vi "Set Component Licenses.vi"(8 "error in (no error)":errorcluster, 10 "License(s)":refnum<class "CycloneDX License.lvclass">[](array[class]), 11 "CycloneDX Component in":refnum<class "CycloneDX Component.lvclass">) -> (0 "error out":errorcluster, 3 "CycloneDX Component out":refnum<class "CycloneDX Component.lvclass">)   [LabVIEW 2017, in "LabVIEW CycloneDX SBOM.lvlib" / "CycloneDX Component.lvclass"]
uses:
  CycloneDX Component.lvclass
  C:/LabVIEW Working Directory/labview-cyclonedx-sbom/Source/CycloneDX/CycloneDX JSON/CycloneDX JSON.lvclass
  CycloneDX License/CycloneDX License.lvclass
  CycloneDX JSON/CycloneDX JSON.lvclass/CycloneDX JSON.ctl
  CycloneDX JSON/Read JSON.vi
  <vilib>/JDP Science/JSONtext/support/Format JSON Array Text.vi
  CycloneDX JSON/CycloneDX JSON.lvclass
  <vilib>/JDP Science/JSONtext/JSONtext.lvlib
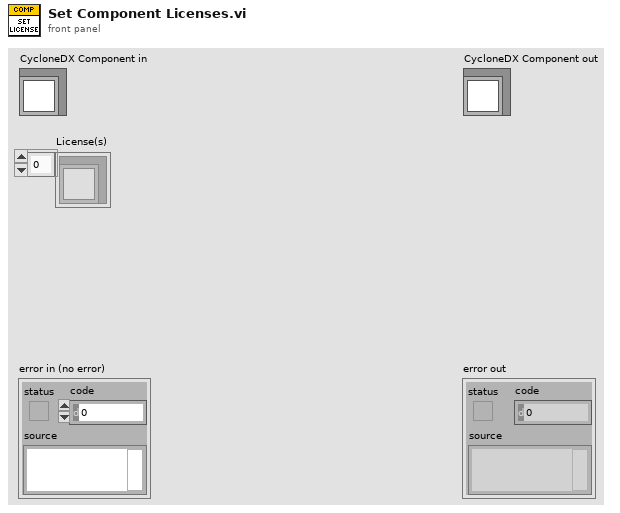
[diagram p1: front panel]
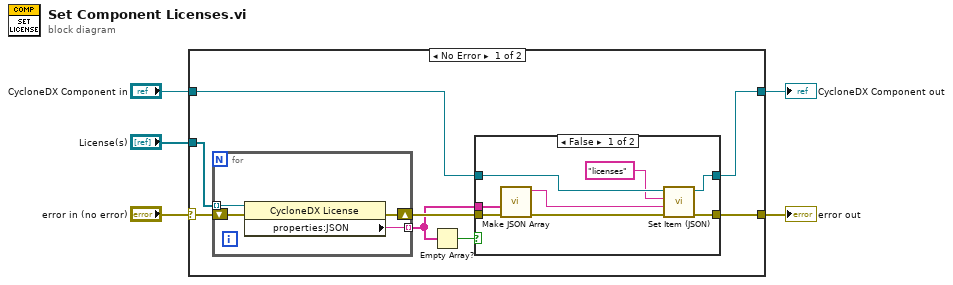
[diagram p0: block diagram]
diagram:
  n1 = case shown="No Error" "error in (no error)" {
    selector: "error in (no error)" -> [w11 w29]
    tunnel: [w8 w29] -> w4
    tunnel: [w9 w28] -> w2
    tunnel: "CycloneDX Component in" -> [w13 w28]
    tunnel: "License(s)" -> [w12 _]
    frame No Error {
      n2 = for {
        tunnel: w12 -> [w27] mode=indexing
        shift-right: [w25] -> w10
        shift-left: w11 -> [w26]
        tunnel: [w24] -> w6 mode=indexing
        n3 = property class="CycloneDX License"(reference=w27, error in=w26) -> (error out=w25:errorcluster, "properties:JSON"=w24:string)  [unwired: 1 out]
      }
      n4 = Empty Array?(array=w6) -> (empty?=w7:bool)
      n5 = case shown="False" w7 {
        tunnel: w13 -> [w21 w22]
        tunnel: w10 -> [w19 w23]
        tunnel: [w17 w22] -> w9
        tunnel: [w16 w23] -> w8
        tunnel: w6 -> [w14 _]
        frame False {
          n6 = call <vilib>:"Make JSON Array.vi"("error in (no error)"=w19, "JSON Elements"=w14) -> ("error out"=w18:errorcluster, "<JSON>"=w15:string)  [unwired: 8 in]
          n7 = call "Set Item (JSON).vi"("error in (no error)"=w18, "JSON to Insert"=w15, "Object (or Item) Path"="licenses", "CycloneDX SBOM in"=w21) -> ("error out"=w16:errorcluster, "CycloneDX SBOM out"=w17:refnum<class "CycloneDX Component.lvclass">)  [unwired: 6 in]
        }
        frame True {
        }
      }
    }
    frame Error {
    }
  }
  "error out" <- w4
  "CycloneDX Component out" <- w2
